vi "SOUR_POW_CORR_COLL_SEN_RCF.vi"(0 "VISA IN":refnum<visa-resource-name>, 1 "Power Meter Channel":string, 2 "Reference Cal Factor(%)":i32, 5 "error in":errorcluster, 7 "Channel":i32) -> (14 "VISA Out":refnum<visa-resource-name>, 19 "error out":errorcluster)   [LabVIEW 2018, in "PNA-X.lvlib"]
doc: "SOURce<cnum>:POWer:CORRection:COLLect:<pmChan>SENsor:RCFactor <num> \n(Read-Write) ) Specifies the reference cal factor for the power sensor connected to channel A or B of \nthe power meter. If the power meter has only a single channel, that channel is considered channel A. \nNote: If the sensor connected to the specified channel of the power meter contains cal factors in \nEPROM (such as the Agilent E-series power sensors), those will be the cal factors used during the \ncalibration sweep. The reference cal factor value associated with this command, and any cal factors \nentered into the PNA for that sensor channel, will not be used. \nParameters \n<cnum> Any existing channel number. If unspecified, value is set to 1 \n<pmChan> Power Meter channel. Choose from: \nA - Channel A \nB - Channel B \n1842\n\n<num> Reference cal factor in percent. Choose any number between 1 and 150. \nExamples SOUR:POW:CORR:COLL:ASEN:RCF 98.7 \nsource1:power2:correction:collect:bsensor:rcfactor 105 \nQuery Syntax SOURce:POWer:CORRection:COLLect:ASENsor:RCFactor? \nSOURce:POWer:CORRection:COLLect:BSENsor:RCFactor? \nReturn Type Numeric \nDefault 100"
uses:
  PNA-X.lvlib
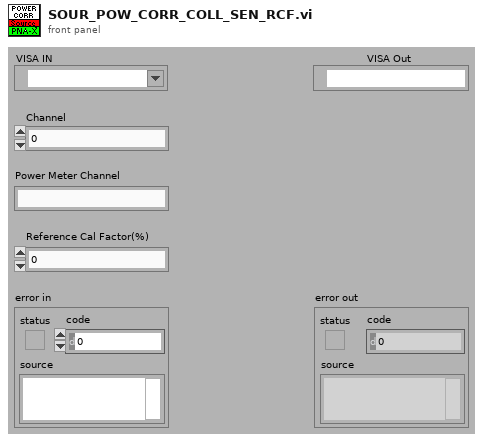
[diagram p1: front panel]
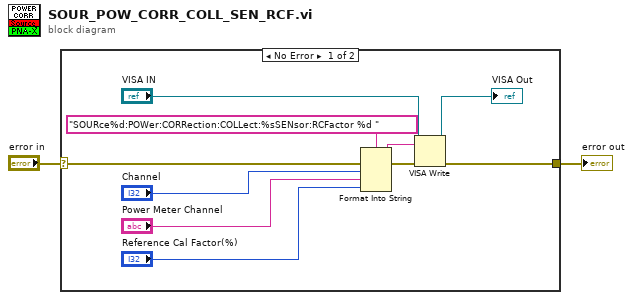
[diagram p0: block diagram]
diagram:
  n1 = case shown="No Error" "error in" {
    selector: "error in" -> [w12 w13]
    tunnel: [w7 w13] -> w1
    frame No Error {
      n2 = Format Into String(format string="SOURce%d:POWer:CORRection:COLLect:%sSENsor:RCFactor %d " ("Cmdline"), error in=w12, "Channel", "Power Meter Channel", "Reference Cal Factor(%)") -> (resulting string=w10:string, error out=w11:errorcluster)  [unwired: 1 in]
      n3 = VISA Write(VISA resource name="VISA IN", write buffer=w10, error in (no error)=w11) -> (VISA resource name out=→"VISA Out":refnum<visa-resource-name>, error out=w7:errorcluster)  [unwired: 1 out]
    }
    frame Error {
    }
  }
  "error out" <- w1
